vi "Warn not supported in GM10.vi"(4 "Source (\"\")":string, 7 "Kind (0: Command)":u16(ring) items=["Command", "Parameter"], 8 "error in (no error)":errorcluster, 11 "VISA resource name":refnum<visa-resource-name>) -> (0 "error out":errorcluster, 3 "VISA resource name out":refnum<visa-resource-name>)   [LabVIEW 2020, in "Yokogawa GX Series.lvlib"]
doc: "This VI logouts from the instrument. Then it can not re-login."
uses:
  <instrlib>/Yokogawa GX Series/Yokogawa GX Series.lvlib
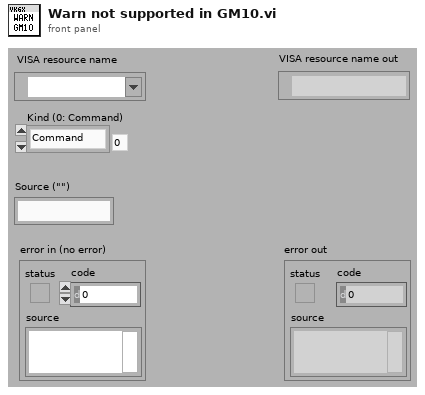
[diagram p1: front panel]
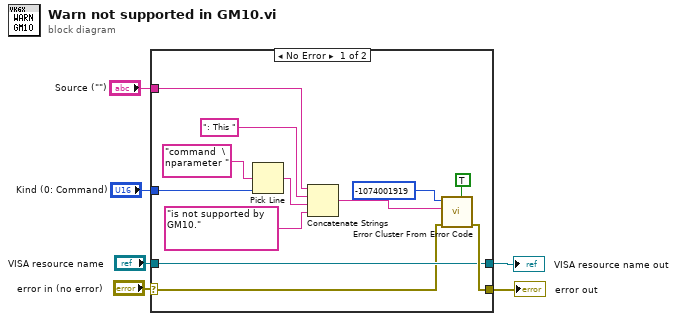
[diagram p0: block diagram]
diagram:
  n1 = case shown="No Error" "error in (no error)" {
    selector: "error in (no error)" -> [w14 w19]
    tunnel: [w16 w19] -> w6
    tunnel: "VISA resource name" -> [w15 w20]
    tunnel: [w15 w20] -> w4
    tunnel: "Kind (0: Command)" -> [w13 _]
    tunnel: "Source (\"\")" -> [w8 _]
    frame No Error {
      n2 = Pick Line(multi-line string="command  \nparameter ", line index=w13) -> (output string=w11:string)  [unwired: 1 in]
      n3 = Concatenate Strings(w8, ": This ", w11, "is not supported by GM10.") -> (w9:string)
      n4 = call <vilib>:"Error Cluster From Error Code.vi"("is warning? (False)"=TRUE, "error in (no error)"=w14, "error message (\"\")"=w9, "error code (0)"=-1074001919) -> ("error out"=w16:errorcluster)  [unwired: 5 in]
    }
    frame Error {
    }
  }
  "error out" <- w6
  "VISA resource name out" <- w4
